vi "VisualizeSiemens.vi"() -> ()   [LabVIEW 2018, in "Visualization.lvlib" / "VisualizeSensor.lvclass"]
doc: "This VI listens for any measurement data associated with the provided PluginName and displays it to the user for analysis. The display is only suitable for data coming from the Siemens Plugin."
uses:
  VisualizeSensor.lvclass
  VisualizeBase/VisualizeBase_class/Requests/clUserEventType.ctl
  <vilib>/event_ctls.llb/usereventprio.ctl
  Sensor/SensorShared/clSensorData.ctl
  <vilib>/Utility/error.llb/Error Cluster From Error Code.vi
  <vilib>/ErrorRing/Error Ring.xnode
  <userlib>/NIST/NISTErrorLib/NISTErrorLib.lvlib
  VisualizeBase/VisualizeBase_class/VisualizeBase.lvclass
  Sensor/SensorShared/SensorShared.lvlib
  Sensor/SensorModule/SensorModule.lvlib
panel:
  out "String Results":string[](array[string])
  in  "Tab Control":enum32{"Chart"}(tab)
  out "Siemens":waveform(dbl)[](graph)=[{"t0"=timestamp(3657200531.6397257 s since 1904-01-01), "dt"=1.0, "Y"=[46.19]}, {"t0"=timestamp(3657200531.6397257 s since 1904-01-01), "dt"=1.0, "Y"=[2.0]}, {"t0"=timestamp(3657200531.6397257 s since 1904-01-01), "dt"=1.0, "Y"=[60.0]}]
  in  "PlotYAxis":u32[](array[numeric])=[0, 1, 0] max=1
  out "Incorrect DataType?":bool
  out "ErrorArray":errorcluster[](array[cluster])
  in  "PluginName":string="Sensor.SiemensDEM0"
  in  "btnStop":bool
  in  "btnReset":bool
  in  "btnClear":bool
  # "0=Left Axis and 1=Right Axis"
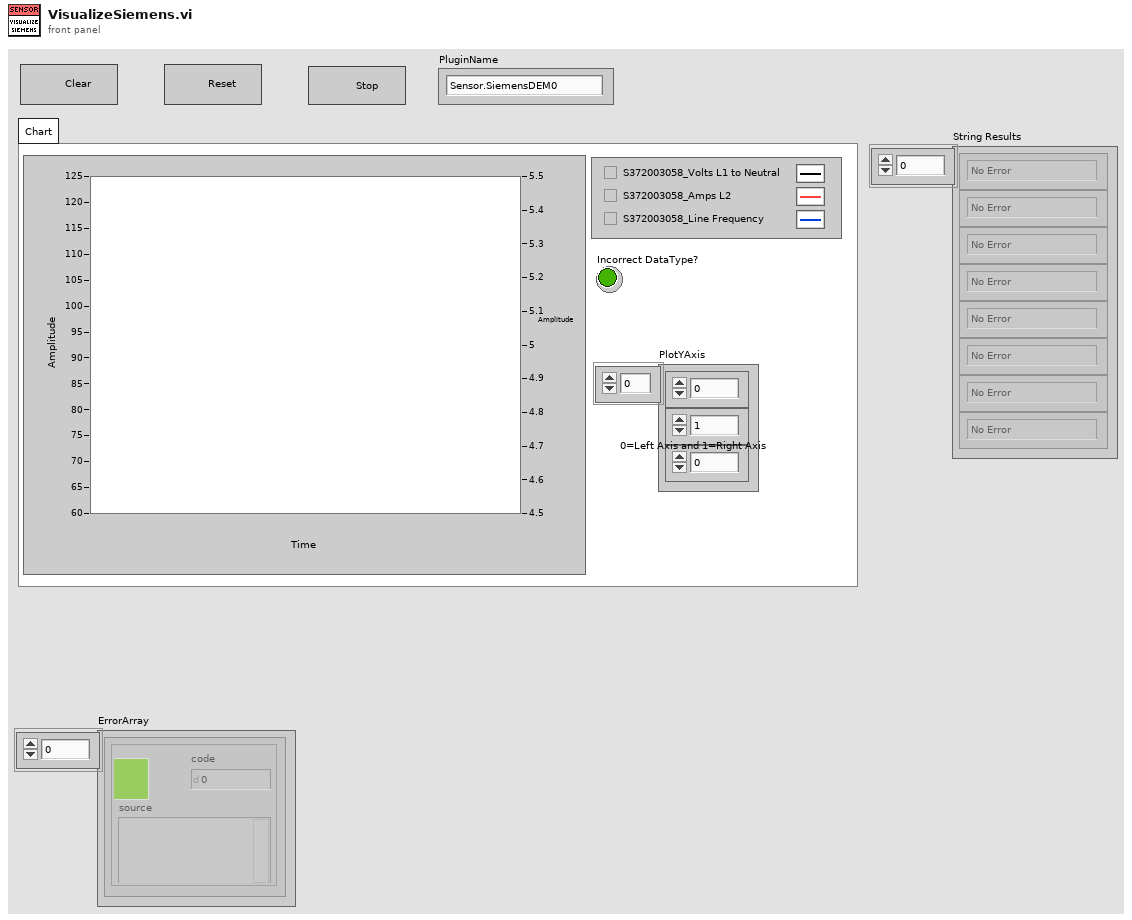
[diagram p1: front panel]
types:
  T1 = typedef "Visualization.lvlib/VisualizeBase.lvclass/clRequestEvents.ctl" = cluster{"StopRequest":refnum<user-event>, "ResetRequest":refnum<user-event>}
  T2 = typedef "SensorShared.lvlib/clBroadcastEvents.ctl" = cluster{"DidInit":refnum<user-event>, "StatusUpdate":refnum<user-event>, "ErrorReport":refnum<user-event>, "DidStop":refnum<user-event>, "PathToINI":refnum<user-event>, "SensorReport":refnum<user-event>, "SensorConfig":refnum<user-event>}
  T3 = typedef "SensorShared.lvlib/clSensorData.ctl" = cluster{"SensorType":string, "SensorData":variant}
  T4 = typedef "Visualization.lvlib/VisualizeBase.lvclass/clUserEventType.ctl" = cluster{"BusIndex":i8, "Data":variant}
  T5 = typedef "usereventprio.ctl" = enum32{"high priority", "normal priority"}
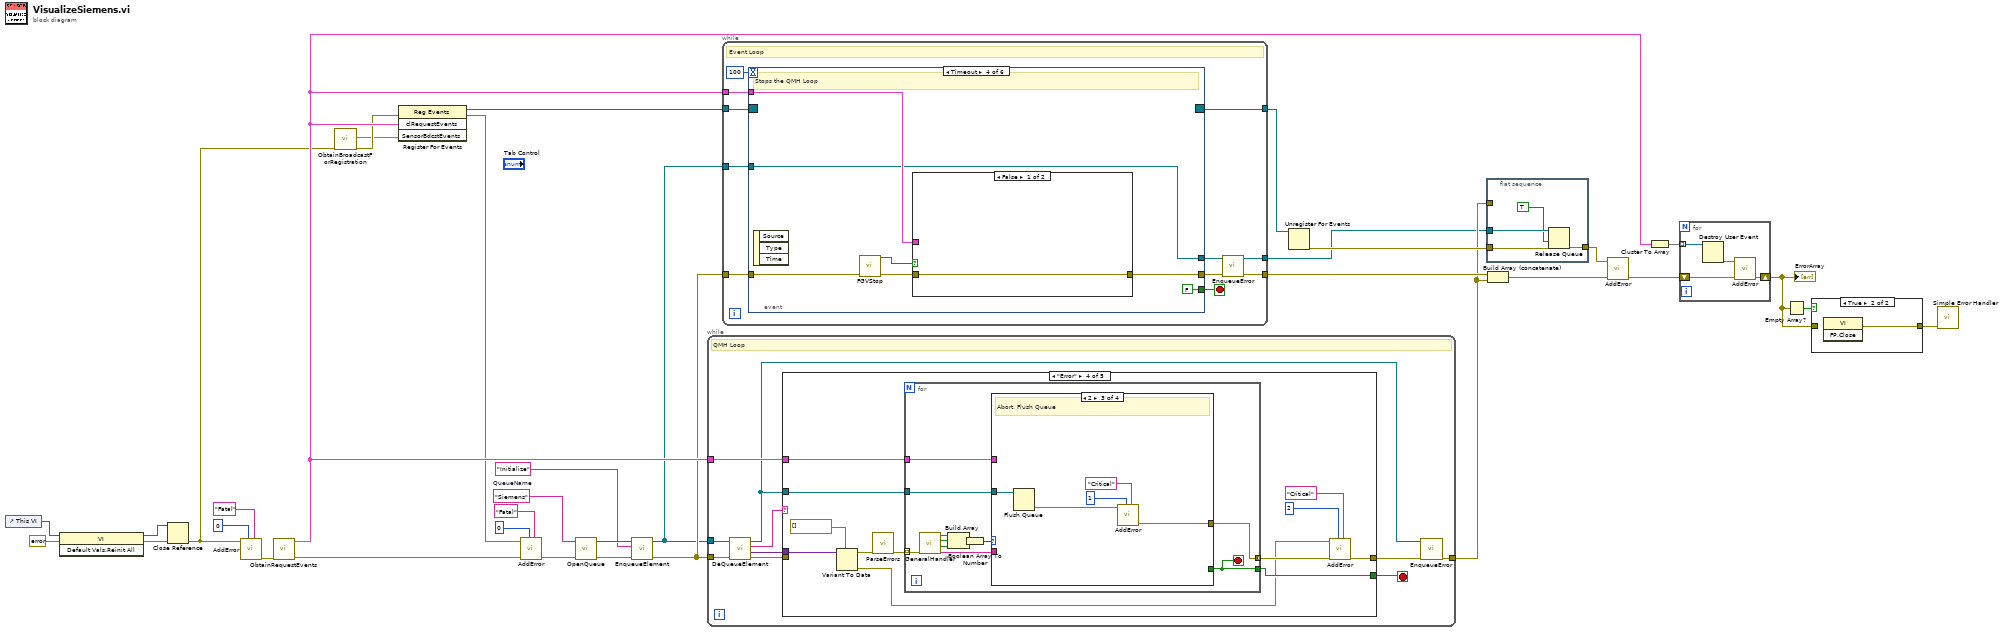
[diagram p0: block diagram]
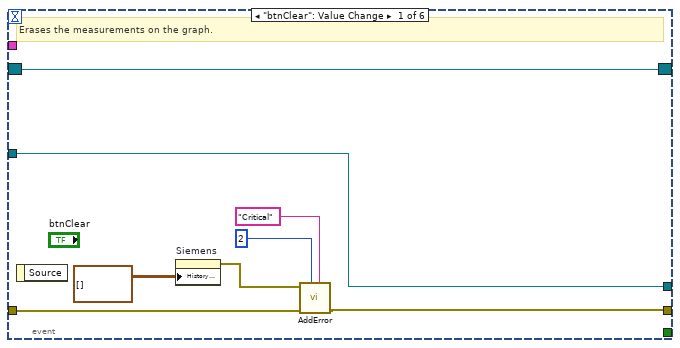
[diagram p2: hidden frame]
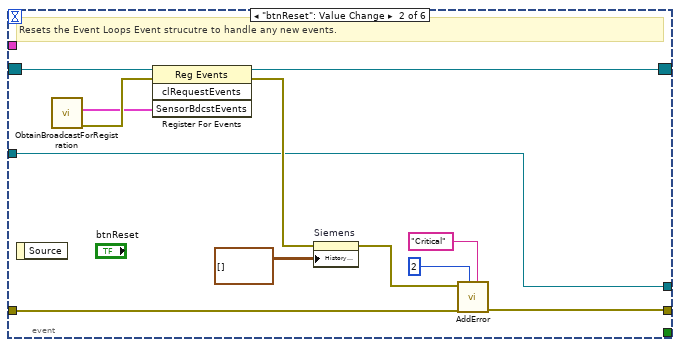
[diagram p3: hidden frame]
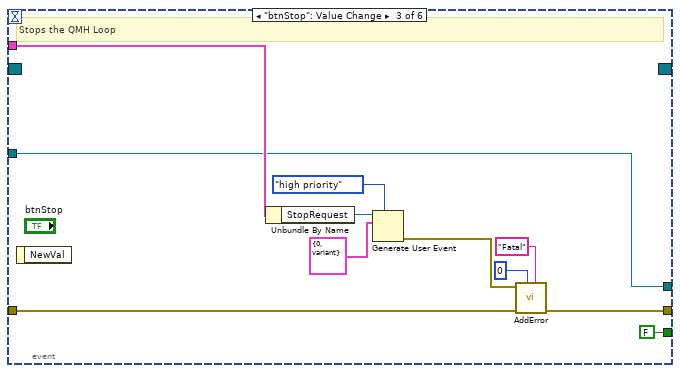
[diagram p4: hidden frame]
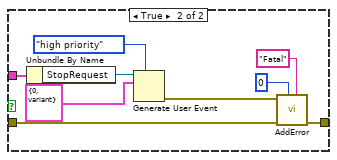
[diagram p5: hidden frame]
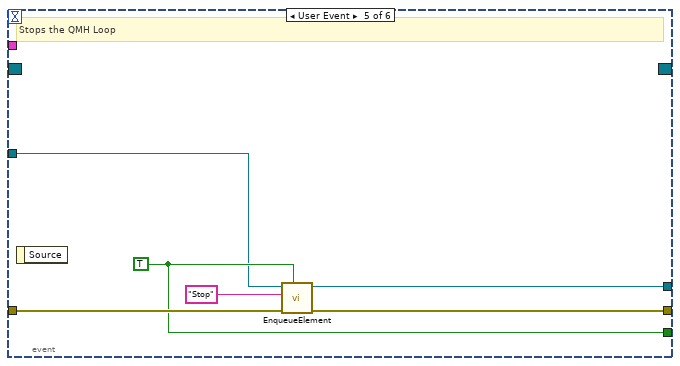
[diagram p6: hidden frame]
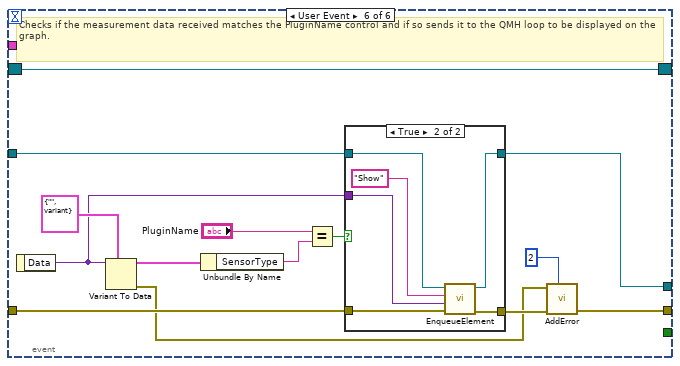
[diagram p7: hidden frame]
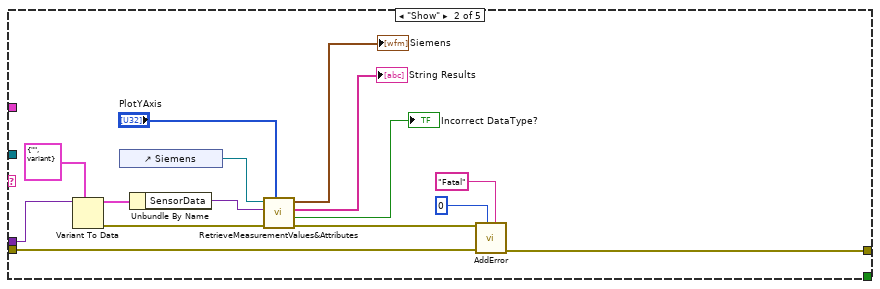
[diagram p10: hidden frame]
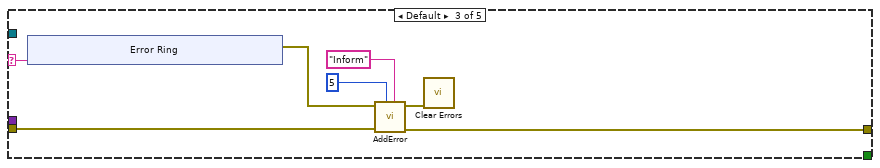
[diagram p11: hidden frame]
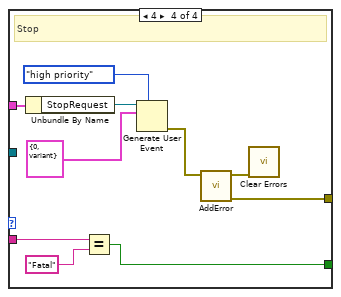
[diagram p14: hidden frame]
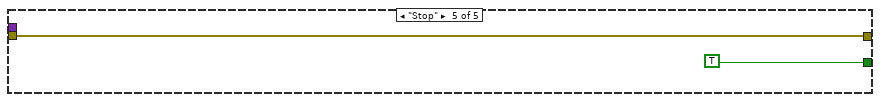
[diagram p15: hidden frame]
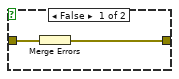
[diagram p16: hidden frame]
diagram:
  w10 = "Siemens"  # QueueName
  n1 = control-ref of="This VI"() -> (w24:refnum<vi>)
  n2 = invoke class="VI" method="Default Vals.Reinit All"(reference=w24, error in=errorcluster {"status"=FALSE, "code"=0, "source"=""} ("error in (no error)")) -> (reference out=w21:refnum<vi>, error out=w22:errorcluster)  [unwired: 1 in, 1 out]
  n3 = Close Reference(reference=w21, error in (no error)=w22) -> (error out=w12:errorcluster)
  n4 = call <userlib>:"AddError.vi"("Severity"="Fatal", "Priority"=u8 0, "error in (no error)"=w12) -> ("ErrorArray"=w34:errorcluster[])  [unwired: 7 in, 1 out]
  n5 = call "ObtainRequestEvents.vi"("Error"=w34) -> ("Error"=w19:errorcluster[], "clRequestEvents"=w26:T1)  [unwired: 9 in]
  n6 = call "ObtainBroadcastForRegistration.vi"("error in (no error)"=w12) -> ("error out"=w13:errorcluster, "SensorBdcstEvents"=w1:T2)  [unwired: 9 in]
  n7 = register-events(error in=w13, w26, w1) -> (reference out=w35:refnum<event-registration>, error out=w17:errorcluster)  [unwired: 1 in]
  n8 = call <userlib>:"AddError.vi"("Severity"="Fatal", "Priority"=u8 0, "ErrorArray"=w19, "error in (no error)"=w17) -> ("ErrorArray"=w11:errorcluster[])  [unwired: 6 in, 1 out]
  n9 = call "OpenQueue.vi"("Error Array In"=w11, "QueueName"=w10) -> ("Error Array Out"=w8:errorcluster[], "queue out"=w9:refnum<queue>)  [unwired: 8 in]
  n10 = call "EnqueueElement.vi"("Error Array In"=w8, "Message"="Initialize", "queue in"=w9) -> ("Error Array Out"=w6:errorcluster[], "queue out"=w5:refnum<queue>)  [unwired: 7 in]
  n11 = while {
    tunnel: w6 -> [w39]
    tunnel: [w42] -> w14
    tunnel: w5 -> [w38]
    tunnel: w26 -> [w44]
    stop <- w45 stop-if-true
    # "QMH Loop"
    n12 = call "DeQueueElement.vi"("Error Array In"=w39, "Queue In"=w38) -> ("Error Array Out"=w37:errorcluster[], "Data"=w40:variant, "Message"=w41:string, "Queue Out"=w36:refnum<queue>)  [unwired: 6 in]
    n13 = case shown="\"Error\"" w41 {
      selector: w41 -> [_ _ w68 _ _]
      tunnel: w40 -> [_ w53 _ w87 _]
      tunnel: w37 -> [w46 w59 w66 _ w114]
      tunnel: [w46 w61 w65 w77 w114] -> w43
      tunnel: [_ _ _ w83 TRUE] -> w45
      tunnel: w44 -> [_ _ _ w82 _]
      tunnel: w36 -> [_ _ _ w81 _]
      frame "Initialize" {
      }
      frame "Show" {
        n14 = Variant To Data(type=T3 {"SensorType"="", "SensorData"=variant} ("clSensorData"), Variant=w53) -> (data=w51:T3, error out=w52:errorcluster)  [unwired: 1 in]
        n15 = control-ref of="Siemens"() -> (w60:refnum<vi>)
        n16 = Unbundle By Name(w51) -> ("SensorData"=w48:variant)
        n17 = call "RetrieveMeasurementValues&Attributes.vi"("PlotYScale"="PlotYAxis", "error in (no error)"=w52, "Variant"=w48, "WaveformChartReference"=w60) -> ("error out"=w55:errorcluster, "Incorrect DataType?"=→"Incorrect DataType?":bool, "Array Of Strings"=→"String Results":string[], "WaveformArrayOut"=→"Siemens":waveform(dbl)[])  [unwired: 4 in]
        n18 = call <userlib>:"AddError.vi"("Severity"="Fatal" ("String"), "Priority"=u8 0, "ErrorArray"=w59, "error in (no error)"=w55) -> ("ErrorArray"=w61:errorcluster[])  [unwired: 6 in, 1 out]
      }
      frame Default {
        n19 = xnode "Error Ring"("parameter 0"=w68) -> ("error out"=w67:errorcluster)
        n20 = call <userlib>:"AddError.vi"("Severity"="Inform" ("String"), "Priority"=u8 5, "ErrorArray"=w66, "error in (no error)"=w67) -> ("ErrorArray"=w65:errorcluster[], "error out"=w64:errorcluster)  [unwired: 6 in]
        n21 = call <vilib>:"Clear Errors.vi"("error in (no error)"=w64) -> ()  [unwired: 5 in, 2 out]
      }
      frame "Error" {
        n22 = Variant To Data(type=errorcluster[] [], Variant=w87) -> (data=w85:errorcluster[], error out=w76:errorcluster)  [unwired: 1 in]
        n23 = call <userlib>:"ParseErrors.vi"("ErrorArray"=w85) -> ("ErrorArray"=w84:errorcluster[])  [unwired: 8 in, 2 out]
        n24 = for {
          tunnel: w84 -> [w98] mode=indexing
          tunnel: [w92] -> w78 mode=concatenating
          tunnel: [w90] -> w83
          tunnel: w82 -> [w89]
          tunnel: w81 -> [w88]
          stop <- w90 stop-if-true
          n25 = call <userlib>:"GeneralHandler.vi"("error in (no error)"=w98) -> ("Severity"=w91:string, "Stop"=w95:bool, "Abort"=w96:bool, "Continue"=w97:bool)  [unwired: 6 in, 1 out]
          n26 = Build Array(w97, w96, w95) -> (w94:bool[])
          n27 = Boolean Array To Number(Boolean array=w94) -> (number=w93:u32)
          n28 = case shown="2" w93 {
            tunnel: [_ _ w103 w112] -> w92
            tunnel: w91 -> [_ _ _ w105]
            tunnel: [_ _ _ w107] -> w90
            tunnel: w89 -> [_ _ _ w106]
            tunnel: w88 -> [_ _ w99 _]
            frame 0, Default {
              # "No Dialog"
            }
            frame 1 {
              # "Continue"
            }
            frame 2 {
              # "Abort, Flush Queue"
              n29 = Flush Queue(queue=w99) -> (error out=w102:errorcluster)  [unwired: 1 in, 2 out]
              n30 = call <userlib>:"AddError.vi"("Severity"="Critical" ("String"), "Priority"=u8 1, "error in (no error)"=w102) -> ("ErrorArray"=w103:errorcluster[])  [unwired: 7 in, 1 out]
            }
            frame 4 {
              # "Stop"
              n31 = Unbundle By Name(w106) -> ("StopRequest"=w113:refnum<user-event>)
              n32 = Equal?(x=w105, y="Fatal" ("x")) -> (x = y?=w107:bool)
              n33 = Generate User Event(priority (normal)=usereventprio."high priority", user event=w113, event data cluster=T4 {"BusIndex"=0, "Data"=variant} ("event data")) -> (error out=w111:errorcluster)  [unwired: 1 in, 1 out]
              n34 = call <userlib>:"AddError.vi"("error in (no error)"=w111) -> ("ErrorArray"=w112:errorcluster[], "error out"=w108:errorcluster)  [unwired: 9 in]
              n35 = call <vilib>:"Clear Errors.vi"("error in (no error)"=w108) -> ()  [unwired: 5 in, 2 out]
            }
          }
        }
        n36 = call <userlib>:"AddError.vi"("Severity"="Critical", "Priority"=u8 2, "ErrorArray"=w78, "error in (no error)"=w76) -> ("ErrorArray"=w77:errorcluster[])  [unwired: 6 in, 1 out]
      }
      frame "Stop" {
      }
    }
    n37 = call "EnqueueError.vi"("Error Array In"=w43, "Queue in"=w36) -> ("Error Array Out"=w42:errorcluster[])  [unwired: 8 in, 1 out]
  }
  n38 = while {
    tunnel: w35 -> [w126]
    tunnel: [w120] -> w31
    tunnel: [w124] -> w33
    tunnel: w26 -> [w123]
    tunnel: w6 -> [w122]
    tunnel: w5 -> [w121]
    tunnel: [w117] -> w4
    stop <- w125 stop-if-true
    # "Event Loop"
    n39 = event shown="[3] Timeout" {
      selector: w126 -> [w128 w146 _ _ _ w189]
      dyn-events: [w128 w145 _ _ _ w189] -> w124
      timeout: 100 -> [_ _ _ _ _ _]
      tunnel: [_ _ FALSE ("Priority? (F)") FALSE ("Priority? (F)") w177 _] -> w125
      tunnel: [w131 w143 w150 w164 w179 w192] -> w119
      tunnel: w123 -> [_ _ w149 w163 _ _]
      tunnel: w122 -> [w132 w144 w157 w160 w180 w193]
      tunnel: w121 -> [w127 w136 w147 w161 w175 w194]
      tunnel: [w127 w136 w147 w161 w178 w190] -> w118
      event "btnClear": Value Change {
        # "Erases the measurements on the graph."
        n40 = event-data() -> ()  [unwired: 1 in, 1 out]
        n41 = property on="Siemens" class="WFChart (strict)"("History Data"=waveform(dbl)[][] []) -> (error out=w130:errorcluster)  [unwired: 2 in, 1 out]
        n42 = call <userlib>:"AddError.vi"("Severity"="Critical", "Priority"=u8 2, "ErrorArray"=w132, "error in (no error)"=w130) -> ("ErrorArray"=w131:errorcluster[])  [unwired: 6 in, 1 out]
      }
      event "btnReset": Value Change {
        # "Resets the Event Loops Event strucutre to handle any new events."
        n43 = event-data() -> ()  [unwired: 1 in, 1 out]
        n44 = call "ObtainBroadcastForRegistration.vi"() -> ("error out"=w137:errorcluster, "SensorBdcstEvents"=w135:T2)  [unwired: 10 in]
        n45 = register-events(reference=w146, error in=w137, w135) -> (reference out=w145:refnum<event-registration>, error out=w139:errorcluster)  [unwired: 1 in]
        n46 = property on="Siemens" class="WFChart (strict)"(error in=w139, "History Data"=waveform(dbl)[][] []) -> (error out=w138:errorcluster)  [unwired: 1 in, 1 out]
        n47 = call <userlib>:"AddError.vi"("Severity"="Critical", "Priority"=u8 2, "ErrorArray"=w144, "error in (no error)"=w138) -> ("ErrorArray"=w143:errorcluster[])  [unwired: 6 in, 1 out]
      }
      event "btnStop": Value Change {
        # "Stops the QMH Loop"
        n48 = event-data() -> ()  [unwired: 1 in, 1 out]
        n49 = Unbundle By Name(w149) -> ("StopRequest"=w155:refnum<user-event>)
        n50 = Generate User Event(priority (normal)=usereventprio."high priority", user event=w155, event data cluster=T4 {"BusIndex"=0, "Data"=variant} ("event data")) -> (error out=w156:errorcluster)  [unwired: 1 in, 1 out]
        n51 = call <userlib>:"AddError.vi"("Severity"="Fatal" ("String"), "Priority"=u8 0, "ErrorArray"=w157, "error in (no error)"=w156) -> ("ErrorArray"=w150:errorcluster[])  [unwired: 6 in, 1 out]
      }
      event Timeout {
        # "Stops the QMH Loop"
        n52 = event-data() -> ()  [unwired: 1 in, 3 out]
        n53 = call "FGVStop.vi"("Error In"=w160) -> ("Error Out"=w158:errorcluster[], "Value"=w159:bool)  [unwired: 9 in]
        n54 = case shown="False" w159 {
          tunnel: w158 -> [w165 w174]
          tunnel: [w165 w167] -> w164
          tunnel: w163 -> [_ w166]
          frame False {
          }
          frame True {
            n55 = Unbundle By Name(w166) -> ("StopRequest"=w172:refnum<user-event>)
            n56 = Generate User Event(priority (normal)=usereventprio."high priority", user event=w172, event data cluster=T4 {"BusIndex"=0, "Data"=variant} ("event data")) -> (error out=w173:errorcluster)  [unwired: 1 in, 1 out]
            n57 = call <userlib>:"AddError.vi"("Severity"="Fatal" ("String"), "Priority"=u8 0, "ErrorArray"=w174, "error in (no error)"=w173) -> ("ErrorArray"=w167:errorcluster[])  [unwired: 6 in, 1 out]
          }
        }
      }
      event User Event {
        w177 = TRUE ("Priority? (F)")
        # "Stops the QMH Loop"
        n58 = event-data() -> ()  [unwired: 1 in, 1 out]
        n59 = call "EnqueueElement.vi"("Priority? (F)"=w177, "Error Array In"=w180, "Message"="Stop", "queue in"=w175) -> ("Error Array Out"=w179:errorcluster[], "queue out"=w178:refnum<queue>)  [unwired: 6 in]
      }
      event User Event {
        # "Checks if the measurement data received matches the PluginName control and if so sends it to the QMH loop to be displayed on the graph."
        n60 = event-data() -> ("Data"=w186:variant)  [unwired: 1 in]
        n61 = Variant To Data(type=T3 {"SensorType"="", "SensorData"=variant} ("clSensorData"), Variant=w186) -> (data=w184:T3, error out=w185:errorcluster)  [unwired: 1 in]
        n62 = Unbundle By Name(w184) -> ("SensorType"=w183:string)
        n63 = Equal?(x="PluginName", y=w183) -> (x = y?=w181:bool)
        n64 = case shown="True" w181 {
          tunnel: [w195 w201] -> w191
          tunnel: w194 -> [w196 w200]
          tunnel: w193 -> [w195 w202]
          tunnel: [w196 w198] -> w190
          tunnel: w186 -> [_ w199]
          frame False {
          }
          frame True {
            n65 = call "EnqueueElement.vi"("Error Array In"=w202, "Data"=w199, "Message"="Show", "queue in"=w200) -> ("Error Array Out"=w201:errorcluster[], "queue out"=w198:refnum<queue>)  [unwired: 6 in]
          }
        }
        n66 = call <userlib>:"AddError.vi"("Priority"=u8 2, "ErrorArray"=w191, "error in (no error)"=w185) -> ("ErrorArray"=w192:errorcluster[])  [unwired: 7 in, 1 out]
      }
    }
    n67 = call "EnqueueError.vi"("Error Array In"=w119, "Queue in"=w118) -> ("Error Array Out"=w120:errorcluster[], "Queue out"=w117:refnum<queue>)  [unwired: 8 in]
  }
  n68 = Unregister For Events(event registration refnum=w33) -> (error out=w30:errorcluster)  [unwired: 1 in]
  n69 = flat-sequence {
    tunnel: w30 -> [w206]
    tunnel: [w205] -> w28
    tunnel: w4 -> [w204]
    tunnel: w14 -> [_]
    frame #0 {
      n70 = Release Queue(queue=w204, force destroy? (F)=TRUE, error in (no error)=w206) -> (error out=w205:errorcluster)  [unwired: 2 out]
    }
  }
  n71 = Build Array (concatenate)(w31, w14) -> (w29:errorcluster[])
  n72 = call <userlib>:"AddError.vi"("ErrorArray"=w29, "error in (no error)"=w28) -> ("ErrorArray"=w27:errorcluster[])  [unwired: 8 in, 1 out]
  n73 = Cluster To Array(cluster=w26) -> (array=w32:refnum<user-event>[])
  n74 = for {
    tunnel: w32 -> [w210] mode=indexing
    shift-right: [w209] -> w3
    shift-left: w27 -> [w208]
    n75 = Destroy User Event(user event=w210) -> (error out=w207:errorcluster)  [unwired: 1 in]
    n76 = call <userlib>:"AddError.vi"("ErrorArray"=w208, "error in (no error)"=w207) -> ("ErrorArray"=w209:errorcluster[])  [unwired: 8 in, 1 out]
  }
  "ErrorArray" <- w3
  n77 = Empty Array?(array=w3) -> (empty?=w25:bool)
  n78 = case shown="True" w25 {
    tunnel: [w211 w213] -> w2
    tunnel: w3 -> [w212 _]
    frame False {
      n79 = Merge Errors(w212) -> (w211:errorcluster)
    }
    frame True {
      n80 = invoke class="VI" method="FP.Close"() -> (error out=w213:errorcluster)  [unwired: 3 in, 2 out]
    }
  }
  n81 = call <vilib>:"Simple Error Handler.vi"("error in (no error)"=w2) -> ()  [unwired: 4 in, 5 out]
